vi "ImagingOrResting.vi"(0 "Scan counters":T1 {"Current part of waveform" items=["Imaging", "Settling", "Resting"]}) -> (1 "Currently at resting part?":bool, 2 "Currently at imaging part?":bool)   [LabVIEW 2010]
uses:
  FPGA_Typedefs/FPGA Scan Counters.ctl
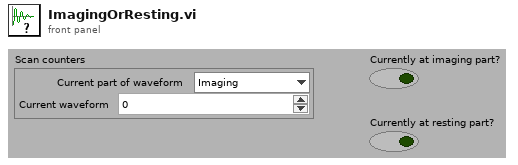
[diagram p1: front panel]
types:
  T1 = typedef "FPGA Scan Counters.ctl" = cluster{"Current part of waveform":u8, "Current waveform":u16}
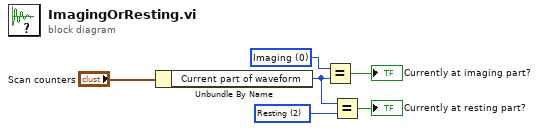
[diagram p0: block diagram]
diagram:
  w6 = u8 0 items=["Imaging", "Settling", "Resting"] ("Current part of waveform")
  w5 = u8 2 items=["Imaging", "Settling", "Resting"] ("Current part of waveform")
  n1 = Unbundle By Name("Scan counters") -> ("Current part of waveform"=w3:u8)
  n2 = Equal?(x=w6, y=w3) -> (x = y?=→"Currently at imaging part?":bool)
  n3 = Equal?(x=w3, y=w5) -> (x = y?=→"Currently at resting part?":bool)
